vi "FetchWave.vi"(8 "error in (no error)":errorcluster caption="错误输入（无错误）", 10 "通道":u16(ring) items=["CH1"=1, "CH2"=2, "CH3"=3, "CH4"=4], 11 "VISA资源名称":refnum<visa-resource-name>) -> (0 "error out":errorcluster caption="错误输出", 2 "波形图":waveform(dbl)(graph), 3 "VISA资源名称 2":refnum<visa-resource-name>)   [LabVIEW 2018]
uses:
  <vilib>/regexp/Match Regular Expression.xnode
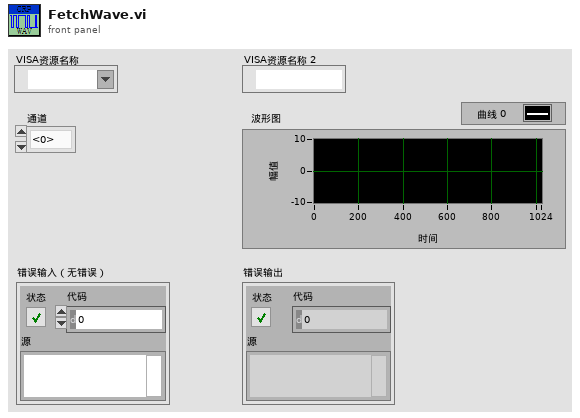
[diagram p1: front panel]
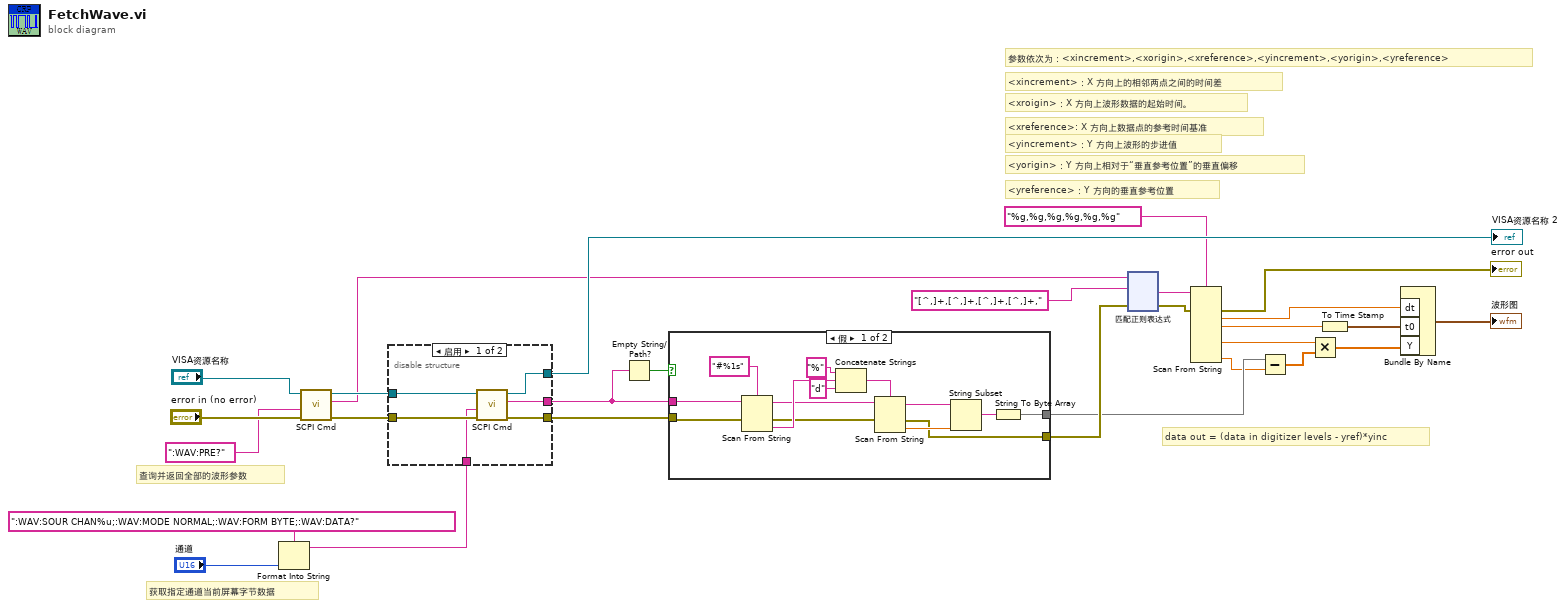
[diagram p0: block diagram]
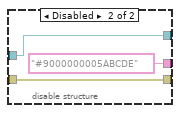
[diagram p3: hidden frame]
diagram:
  # "获取指定通道当前屏幕字节数据"
  # "data out = (data in digitizer levels - yref)*yinc"
  # "<yreference>：Y 方向的垂直参考位置"
  # "<xreference>: X 方向上数据点的参考时间基准"
  # "<yorigin>：Y 方向上相对于“垂直参考位置”的垂直偏移"
  # "<yincrement>：Y 方向上波形的步进值"
  # "<xroigin>：X 方向上波形数据的起始时间。"
  # "<xincrement>：X 方向上的相邻两点之间的时间差"
  # "参数依次为：<xincrement>,<xorigin>,<xreference>,<yincrement>,<yorigin>,<yreference>"
  # "查询并返回全部的波形参数"
  n1 = Format Into String(format string=":WAV:SOUR CHAN%u;:WAV:MODE NORMAL;:WAV:FORM BYTE;:WAV:DATA?" ("格式字符串"), "通道") -> (resulting string=w27:string)  [unwired: 2 in, 1 out]
  n2 = call "SCPI Cmd.vi"("VISA资源名称"="VISA资源名称", "SCPI字符串"=":WAV:PRE?", "错误输入（无错误）"="error in (no error)") -> ("VISA资源名称输出"=w22:refnum<visa-resource-name>, "读取缓冲区"=w13:string, "错误输出"=w19:errorcluster)  [unwired: 4 in, 1 out]
  n3 = disable-structure shown="启用" {
    disable-tunnel: w19 -> [w34 w37]
    disable-tunnel: w27 -> [w33 _]
    disable-tunnel: [w32 "#9000000005ABCDE" ("读取缓冲区")] -> w25
    disable-tunnel: [w31 w37] -> w26
    disable-tunnel: w22 -> [w30 w35]
    disable-tunnel: [w29 w35] -> w23
    frame Enabled {
      n4 = call "SCPI Cmd.vi"("VISA资源名称"=w30, "SCPI字符串"=w33, "错误输入（无错误）"=w34) -> ("VISA资源名称输出"=w29:refnum<visa-resource-name>, "读取缓冲区"=w32:string, "错误输出"=w31:errorcluster)  [unwired: 4 in, 1 out]
    }
    frame Disabled {
    }
  }
  "VISA资源名称 2" <- w23
  n5 = Empty String/Path?(string/path=w25) -> (empty?=w24:bool)
  n6 = case shown="假" w24 {
    tunnel: w26 -> [w51 w52]
    tunnel: [w38 w52] -> w12
    tunnel: [w39 _] -> w11
    tunnel: w25 -> [w40 _]
    frame False {
      n7 = Scan From String(format string="#%1s" ("格式字符串"), input string=w40, error in=w51) -> (remaining string=w46:string, error out=w41:errorcluster, output 1=w49:string)  [unwired: 2 in, 1 out]
      n8 = Concatenate Strings("%" ("字符串"), w49, "d" ("字符串")) -> (w45:string)
      n9 = Scan From String(format string=w45, input string=w46, error in=w41) -> (remaining string=w44:string, error out=w38:errorcluster, output 1=w43:dbl)  [unwired: 2 in, 1 out]
      n10 = String Subset(string=w44, length (rest)=w43) -> (substring=w42:string)  [unwired: 1 in]
      n11 = String To Byte Array(string=w42) -> (unsigned byte array=w39:u8[])
    }
    frame True {
    }
  }
  n12 = xnode "匹配正则表达式"("输入字符串"=w13, "正则表达式"="[^,]+,[^,]+,[^,]+,[^,]+,", "错误输入"=w12) -> ("匹配之后"=w14:string, "错误输出"=w2:errorcluster)  [unwired: 3 in, 3 out]
  n13 = Scan From String(format string="%g,%g,%g,%g,%g,%g" ("格式字符串"), input string=w14, error in=w2) -> (error out=→"error out":errorcluster, output 1=w5:dbl, output 2=w6:dbl, output 4=w9:dbl, output 6=w10:dbl)  [unwired: 9 in, 2 out]
  n14 = Subtract(x=w11, y=w10) -> (x-y=w8:dbl[])
  n15 = Multiply(x=w9, y=w8) -> (x*y=w7:dbl[])
  n16 = To Time Stamp(1:w6) -> (0:w4:timestamp)
  n17 = Bundle By Name("dt"=w5, "t0"=w4, "Y"=w7) -> (→"波形图":waveform(dbl))  [unwired: 1 in]
